vi "Read Setting.vi"(8 "error in (no error)":errorcluster, 10 "Tag Name":string, 11 "Save Restore Settings in":refnum<class "Save Restore Settings.lvclass">) -> (0 "error out":errorcluster, 1 "Tag Attribute":variant, 3 "Save Restore Settings out":refnum<class "Save Restore Settings.lvclass">)   [LabVIEW 2016, in "Save Restore Settings.lvclass"]
uses:
  <userlib>/_MGI/Application Control/MGI Save Restore Settings/Save Restore Settings.lvclass
  <userlib>/_MGI/Application Control/MGI Save Restore Settings/Save Restore Settings.lvclass/Save Restore Settings.ctl
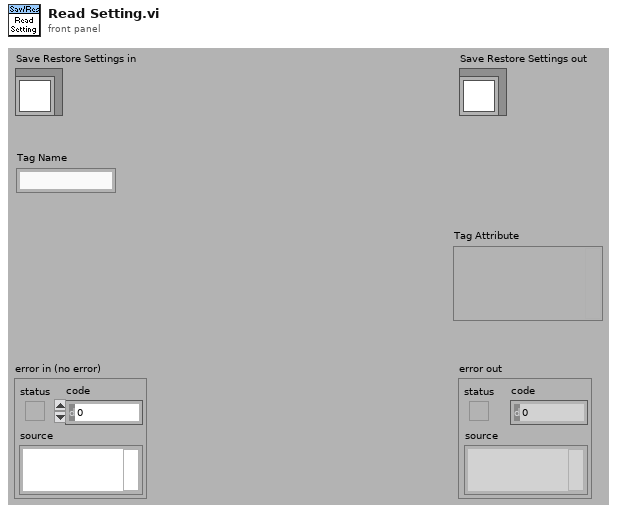
[diagram p1: front panel]
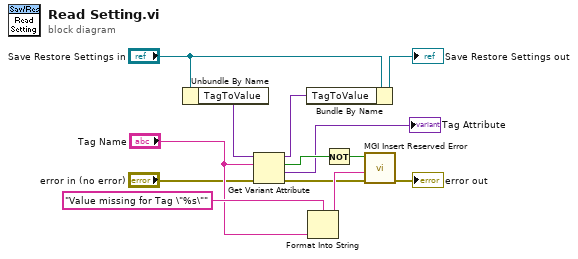
[diagram p0: block diagram]
diagram:
  n1 = Unbundle By Name("Save Restore Settings in") -> ("TagToValue"=w8:variant)
  n2 = Get Variant Attribute(Variant=w8, name="Tag Name", error in="error in (no error)") -> (duplicate Variant=w4:variant, found=w3:bool, value=→"Tag Attribute":variant, error out=w5:errorcluster)  [unwired: 1 in]
  n3 = Bundle By Name(cluster="Save Restore Settings in", "TagToValue"=w4) -> (→"Save Restore Settings out":refnum<class "Save Restore Settings.lvclass">)
  n4 = Format Into String(format string="Value missing for Tag \"%s\"", "Tag Name") -> (resulting string=w10:string)  [unwired: 2 in, 1 out]
  n5 = Not(x=w3) -> (.not. x?=w2:bool)
  n6 = call <userlib>:"MGI Insert Reserved Error.vi"("Error In"=w5, "Error Description"=w10, "Error? (T)"=w2) -> ("Error Out"=→"error out":errorcluster)  [unwired: 8 in]
